vi "mock_v1.vi"() -> ()   [LabVIEW 2022 SP3]
panel:
  in  "Up":bool
  in  "Down":bool
  in  "Forward":bool
  in  "Left":bool
  in  "Backward":bool
  in  "Right":bool
  in  "STOP":bool
  in  "ON/OFF":bool
  in  "Baud Rate":dbl
  in  "Port COM:":tag
  in  "Z Axis":dbl
  in  "Y Axis":dbl
  in  "X Axis":dbl
  # "Movement"
  # "Directional Pad"
  # "Communication"
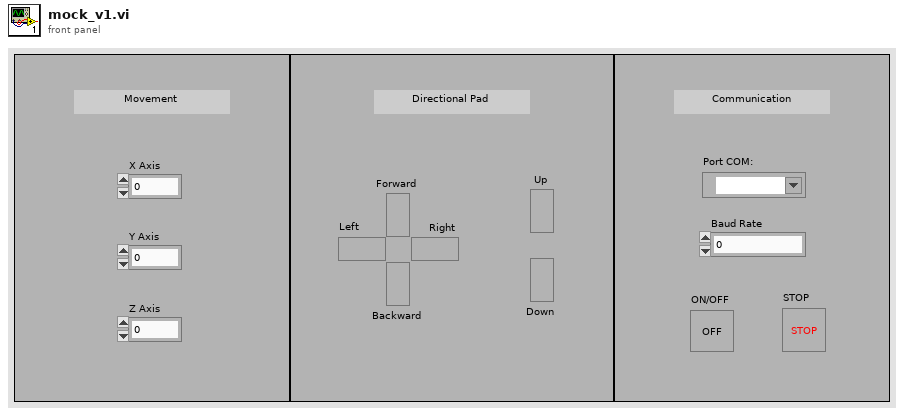
[diagram p1: front panel]
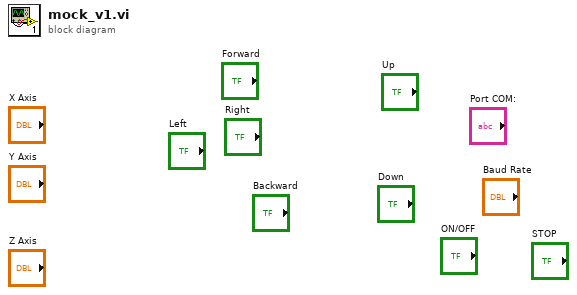
[diagram p0: block diagram]
diagram:
